vi "isBlockOn.vi"(8 "error in (no error)":errorcluster) -> (0 "error out":errorcluster, 2 "block on 2":bool, 3 "block on 1":bool)   [LabVIEW 2015, in "ESLSCDLL.lvlib"]
uses:
  ESLSCDLL.lvlib
  Globals.vi
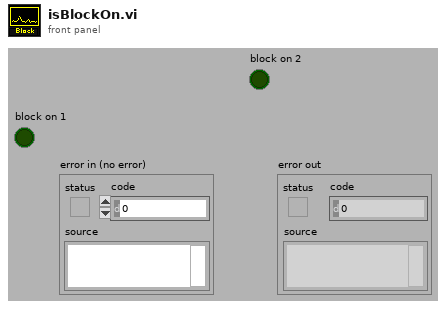
[diagram p1: front panel]
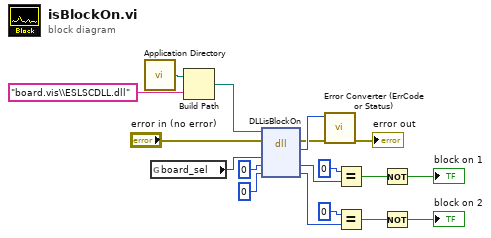
[diagram p0: block diagram]
diagram:
  n1 = call <vilib>:"Application Directory.vi"() -> ("Application Directory"=w7:path)
  n2 = global read "Globals.vi" "board_sel"() -> (w1:u32)
  n3 = Build Path(base path=w7, name or relative path="board.vis\\ESLSCDLL.dll") -> (appended path=w5:path)
  n4 = dll-call lib="C:/ENTW/PCIE/LV64/board.vis/ESLSCDLL.dll" fn="DLLisBlockOn" ("lwlscdll.dll:DLLWriteLongS0")(path in=w5, error in="error in (no error)", "board_sel"=w1, "blockOn0"=u8 0 ("blockOn"), "blockOn1"=u8 0) -> (error out=w10:errorcluster, "es_status_codes"=w11:i32, "blockOn0"=w15:u8, "blockOn1"=w2:u8)  [unwired: 2 in, 1 out]
  n5 = call "Error Converter (ErrCode or Status).vi"("error in (no error)"=w10, "error code"=w11) -> ("error out"=→"error out":errorcluster)  [unwired: 9 in]
  n6 = Equal?(x=u8 0, y=w15) -> (x = y?=w17:bool)
  n7 = Equal?(x=u8 0, y=w2) -> (x = y?=w13:bool)
  n8 = Not(x=w17) -> (.not. x?=→"block on 1":bool)
  n9 = Not(x=w13) -> (.not. x?=→"block on 2":bool)
